vi "Teleop.vi"(10 "Match Info":T2={"Autonomous Elapsed Seconds"=0.0, "TeleOp Elapsed Seconds"=0.0, "Disabled Elapsed Seconds"=0.0, "Visited Autonomous"=FALSE, "Visited TeleOp"=FALSE, "Visited Disabled"=FALSE, "Autonomous Settings"={"Autonomous Style"=enum."Independent", "VI Refnum"=refnum}}, 11 "Call Context":T3) -> ()   [LabVIEW 2020]
doc: "This VI is called for each enabled TeleOp packet received from the DS. It is typically used to read from joysticks and other inputs and update I/O or setpoints for timed control loops. It should complete and return within 20 milliseconds or risk missing DS packets."
uses:
  <vilib>/Rock Robotics/WPI/DriverStation/WPI_DriverStationDerivedRobotMode.ctl
  <vilib>/Rock Robotics/WPI/DriverStation/WPI_DriverStationMatch Info.ctl
  Drive/Implementation/Robot Velocities.ctl
  <vilib>/Rock Robotics/WPI/Joystick/XBox Axes Indexer.ctl
  Drive/Implementation/Driving Mode.ctl
  <vilib>/Rock Robotics/WPI/Joystick/XBox Buttons Indexer.ctl
  97e635d3-2ee8-4cef-b098-8ad6758c7b24.vi
  <vilib>/Rock Robotics/WPI/Utilities/WPI_GetSetVariantRefNum.vi
  <vilib>/Rock Robotics/WPI/ThirdParty/Phoenix-LabVIEW/Pigeon IMU/CTRE_PigeonIMU_GetYPR.vi
panel:
  in  "Max Velocities":T1={"vx"=10.0, "vy"=10.0, "w"=180.0}
  in  "Deadband":dbl=0.1
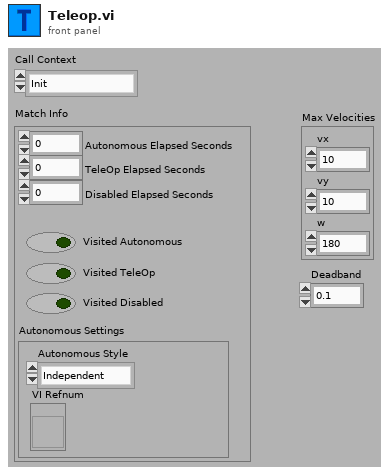
[diagram p1: front panel]
types:
  T1 = typedef "Robot Velocities.ctl" = cluster{"vx":dbl, "vy":dbl, "w":dbl}
  T2 = typedef "WPI_DriverStationMatch Info.ctl" = cluster{"Autonomous Elapsed Seconds":dbl, "TeleOp Elapsed Seconds":dbl, "Disabled Elapsed Seconds":dbl, "Visited Autonomous":bool, "Visited TeleOp":bool, "Visited Disabled":bool, "Autonomous Settings":cluster{"Autonomous Style":enum16{"Iterative", "Independent"}, "VI Refnum":refnum<vi>}}
  T3 = typedef "WPI_DriverStationDerivedRobotMode.ctl" = enum16{"Init", "Execute", "Stop"}
  T4 = typedef "XBox Buttons Indexer.ctl" = enum16{"A", "B", "X", "Y", "Left Bumper", "Right Bumper", "Back", "Start", "Left Joystick", "Right Joystick"}
  T5 = typedef "Driving Mode.ctl" = enum16{"Robot Centric", "Field Centric"}
  T6 = typedef "XBox Axes Indexer.ctl" = enum16{"Left X", "Left Y", "Left Trigger", "Right Trigger", "Right X", "Right Y"}
  T7 = typedef "WPI_JoystickDevRef.ctl" = cluster{"Device":T8}
  T8 = typedef "WPI_JoystickDeviceEnum.ctl" = enum16{"USB 0", "USB 1", "USB 2", "USB 3", "USB 4", "USB 5"}
  T9 = typedef "CTRE_PigeonIMU_DeviceRef.ctl" = cluster{"DeviceStatus":errorcluster, "Device Number":u8, "Type":T10, "Device ID":u32, "Handle":u64, "UsageFrame":u32, "Library Path":path}
  T10 = typedef "CTRE_PigeonIMU_ConnectionType.ctl" = u32
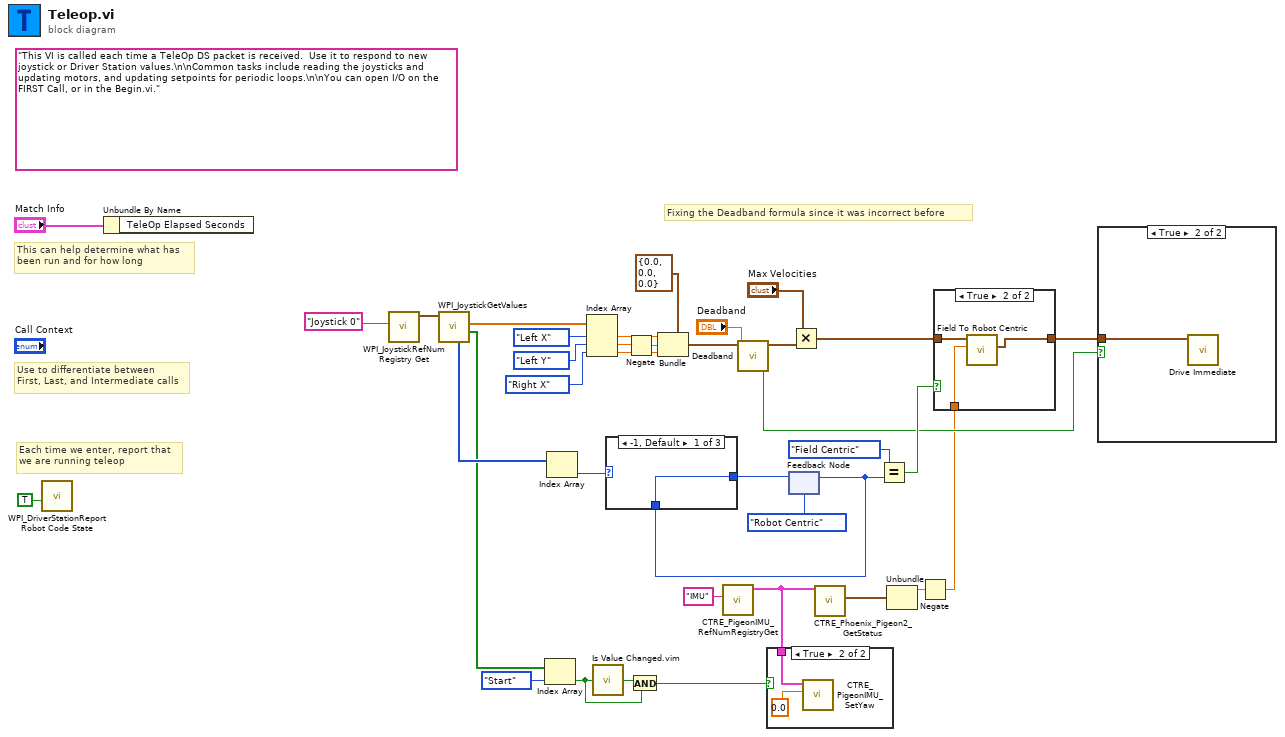
[diagram p0: block diagram]
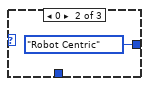
[diagram p4: hidden frame]
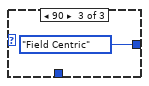
[diagram p5: hidden frame]
diagram:
  (unwired) "This VI is called each time a TeleOp DS packet is received.  Use it to respond to new joystick or Driver Station values.\n\nCommon tasks include reading the joysticks and updating motors, and updating setpoints for periodic loops.\n\nYou can open I/O on the FIRST Call, or in the Begin.vi."
  # "Fixing the Deadband formula since it was incorrect before"
  # "Each time we enter, report that\nwe are running teleop"
  # "Use to differentiate between\nFirst, Last, and Intermediate calls"
  # "This can help determine what has\nbeen run and for how long"
  n1 = call <vilib>:"WPI_DriverStationReport Robot Code State.vi"("TeleOp"=TRUE ("Autonomous")) -> ()  [unwired: 10 in, 1 out]
  n2 = Unbundle By Name("Match Info") -> ()  [unwired: 1 out]
  n3 = call <vilib>:"WPI_JoystickRefNum Registry Get.vi"("refnum name"="Joystick 0") -> ("JoystickDevRef"=w34:T7)  [unwired: 1 in, 9 out]
  n4 = call <vilib>:"WPI_JoystickGetValues.vi"("JoystickDevRef"=w34) -> ("Buttons"=w11:bool[], "Axes"=w33:dbl[], "POVs"=w21:i16[])  [unwired: 6 in, 2 out]
  n5 = Index Array(array=w11, index=XBox_Buttons_Indexer."Start" ("XBox Buttons")) -> (element=w8:bool)
  n6 = Index Array(array=w21) -> (element=w20:i16)  [unwired: 1 in]
  n7 = Index Array(array=w33, index #1=XBox_Axes_Indexer."Left X" ("XBox Axes"), index #2=XBox_Axes_Indexer."Left Y" ("XBox Axes"), index #3=XBox_Axes_Indexer."Right X" ("XBox Axes")) -> (element #1=w29:dbl, element #2=w4:dbl, element #3=w28:dbl)
  n8 = call "Is Value Changed.vim"("value"=w8) -> ("changed or first call?"=w9:bool)
  n9 = Negate(x=w4) -> (-x=w3:dbl)
  n10 = And(x=w9, y=w8) -> (x .and. y?=w7:bool)
  n11 = Bundle(cluster=T1 {"vx"=0.0, "vy"=0.0, "w"=0.0} ("Robot Velocities"), "vx"=w29, "vy"=w3, "w"=w28) -> (w26:T1)
  n12 = call <vilib>:"CTRE_PigeonIMU_RefNumRegistryGet.vi"("refnum name"="IMU") -> ("PigeonIMUDevRef"=w6:T9)  [unwired: 9 in, 1 out]
  n13 = call "Deadband.vi"("Deadband"="Deadband", "Robot Velocities"=w26) -> ("Sending Input?"=w5:bool, "Adjusted Robot Velocities"=w24:T1)  [unwired: 8 in]
  n14 = case shown="True" w7 {
    tunnel: w6 -> [_ w38]
    frame False {
    }
    frame True {
      n15 = call <vilib>:"CTRE_PigeonIMU_SetYaw.vi"("Value"=0.0, "PigeonIMUDevRef"=w38) -> ()  [unwired: 8 in, 2 out]
    }
  }
  n16 = feedback #1(Driving_Mode."Robot Centric") -> (w18:T5)
  n17 = case shown="-1, Default" w20 {
    tunnel: [w40 Driving_Mode."Robot Centric" Driving_Mode."Field Centric"] -> w19
    tunnel: w18 -> [w40 _ _]
    frame -1, Default {
    }
    frame 0 {
    }
    frame 90 {
    }
  }
  n18 = feedback-in #1(w19) -> ()
  n19 = Multiply(x="Max Velocities", y=w24) -> (x*y=w15:T1)
  n20 = call-poly <vilib>:"CTRE_Phoenix_Pigeon2_GetStatus.vi"("PigeonIMUDevRef"=w6) -> ("Yaw Pitch Roll"=w13:cluster{"Yaw":dbl, "Pitch":dbl, "Roll":dbl})  [unwired: 8 in, 2 out]
  n21 = Equal?(x=Driving_Mode."Field Centric", y=w18) -> (x = y?=w16:bool)
  n22 = Unbundle(w13) -> ("Yaw"=w2:dbl)  [unwired: 2 out]
  n23 = Negate(x=w2) -> (-x=w1:dbl)
  n24 = case shown="True" w16 {
    tunnel: w15 -> [w43 w46]
    tunnel: [w43 w45] -> w14
    tunnel: w1 -> [_ w44]
    frame False {
    }
    frame True {
      n25 = call "Field To Robot Centric.vi"("IMU Value (offset)"=w44, "Robot Velocities"=w46) -> ("Robot Centric Velocities"=w45:T1)  [unwired: 8 in, 1 out]
    }
  }
  n26 = case shown="True" w5 {
    tunnel: w14 -> [_ w47]
    frame False {
    }
    frame True {
      n27 = call "Drive Immediate.vi"("Robot Velocities"=w47) -> ()  [unwired: 10 in, 1 out]
    }
  }
